vi "SSI_Frequency Bandwidth.vi"(2 "Frequency":dbl, 3 "Instrument Mode":T1(ring)) -> (0 "Output":dbl)   [LabVIEW 2011]
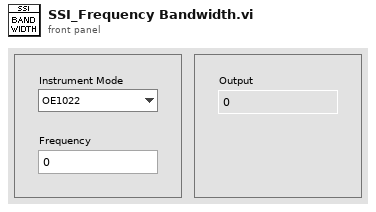
[diagram p1: front panel]
types:
  T1 = enum16{"OE1022", "OE1022D", "OE1201", "OE1311", "OE1351", "OE1301", "OE2031-10M", "OE2041-30M", "OE2041-60M", "OE2052", "OE2011&OE2012", "OE2021&OE2022"}
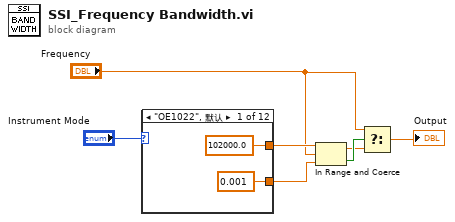
[diagram p0: block diagram]
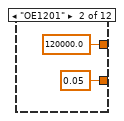
[diagram p2: hidden frame]
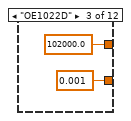
[diagram p3: hidden frame]
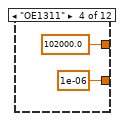
[diagram p4: hidden frame]
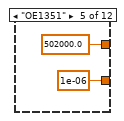
[diagram p5: hidden frame]
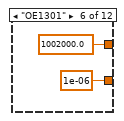
[diagram p6: hidden frame]
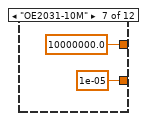
[diagram p7: hidden frame]
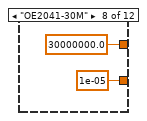
[diagram p8: hidden frame]
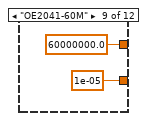
[diagram p9: hidden frame]
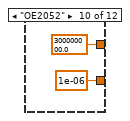
[diagram p10: hidden frame]
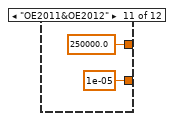
[diagram p11: hidden frame]
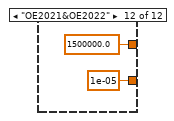
[diagram p12: hidden frame]
diagram:
  n1 = case shown="\"OE1022\", 默认" "Instrument Mode" {
    tunnel: [102000.0 120000.0 102000.0 102000.0 502000.0 1002000.0 10000000.0 30000000.0 60000000.0 300000000.0 250000.0 1500000.0] -> w6
    tunnel: [0.001 0.05 0.001 1e-06 1e-06 1e-06 1e-05 1e-05 1e-05 1e-06 1e-05 1e-05] -> w5
    frame "OE1022", Default {
    }
    frame "OE1201" {
    }
    frame "OE1022D" {
    }
    frame "OE1311" {
    }
    frame "OE1351" {
    }
    frame "OE1301" {
    }
    frame "OE2031-10M" {
    }
    frame "OE2041-30M" {
    }
    frame "OE2041-60M" {
    }
    frame "OE2052" {
    }
    frame "OE2011&OE2012" {
    }
    frame "OE2021&OE2022" {
    }
  }
  n2 = In Range and Coerce(upper limit=w6, x="Frequency", lower limit=w5) -> (coerced(x)=w3:dbl, In Range?=w7:bool)
  n3 = Select(t="Frequency", s=w7, f=w3) -> (s? t:f=→"Output":dbl)
